vi "Init Minesweeper Drawing Events.vi"(8 "Error In":errorcluster) -> (0 "Error Out":errorcluster, 2 "user event out":refnum<user-event>, 3 "Event Registration Refnum":refnum<event-registration>)   [LabVIEW 2011]
uses:
  Minesweeper Drawing Event Type Def.ctl
  Minesweeper Drawing Operation Type Def.ctl
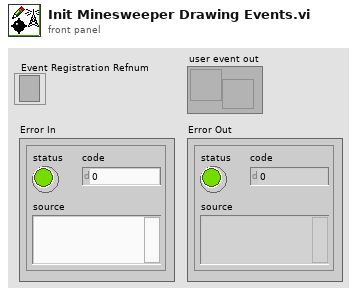
[diagram p1: front panel]
types:
  T1 = typedef "Minesweeper Drawing Event Type Def.ctl" = cluster{"Minesweeper Drawing Operation":T2, "Operation Index (row, column)":cluster{"x":i16, "y":i16}}
  T2 = typedef "Minesweeper Drawing Operation Type Def.ctl" = enum16{"Initialize", "Uncover", "Flag", "Unflag"}
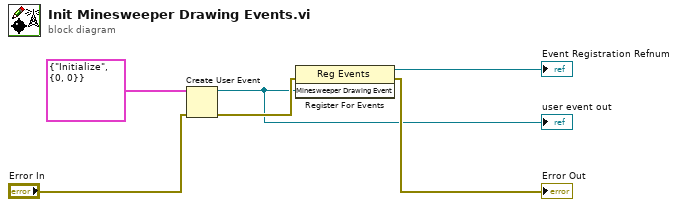
[diagram p0: block diagram]
diagram:
  n1 = Create User Event(user event datatype=T1 {"Minesweeper Drawing Operation"=enum."Initialize", "Operation Index (row, column)"={"x"=0, "y"=0}} ("Minesweeper Drawing Event"), error in="Error In") -> (user event=w1:refnum<user-event>, error out=w4:errorcluster)
  "user event out" <- w1
  n2 = register-events(error in=w4, w1) -> (reference out=→"Event Registration Refnum":refnum<event-registration>, error out=→"Error Out":errorcluster)  [unwired: 1 in]
